vi "Log In.vi"(0 "SLSC Remote in":refnum<class "SLSC Remote.lvclass">, 1 "username":string, 2 "password":string, 5 "chassis":refnum<k21>, 11 "error in (no error)":errorcluster, 12 "connect timeout (60 sec)":dbl=60.0, 13 "save credentials to disk? (F)":bool) -> (4 "SLSC Remote out":refnum<class "SLSC Remote.lvclass">, 15 "error out":errorcluster)   [LabVIEW 2015, in "SLSC Interfaces.lvlib" / "SLSC Remote.lvclass"]
uses:
  SLSC Remote.lvclass
  <vilib>/NI/NI JSONRPC Server Framework/Classes/Server/JSONRPC Server.lvclass
  <vilib>/rajsite/i3-json/i3-json.lvlib
  <vilib>/rajsite/i3-json/JSON Generation/Create Value Files/Create Value - Object.vi
  <vilib>/rajsite/i3-json/JSON Generation/Add Object Parameter Files/Add Object Parameter - String.vi
  <vilib>/httpClient/LabVIEWHTTPClient.lvlib
  <vilib>/NI/NI JSONRPC Server Framework/Classes/Server/Format Client Request (Auto-Increment).vi
  <vilib>/httpClient/POSTBuffer.vi
  <vilib>/rajsite/i3-json/JSON Generation/Add Object Parameter Files/Add Object Parameter - Numeric.vi
  <vilib>/rajsite/i3-json/JSON Generation/Add Object Parameter Files/Add Object Parameter - Boolean.vi
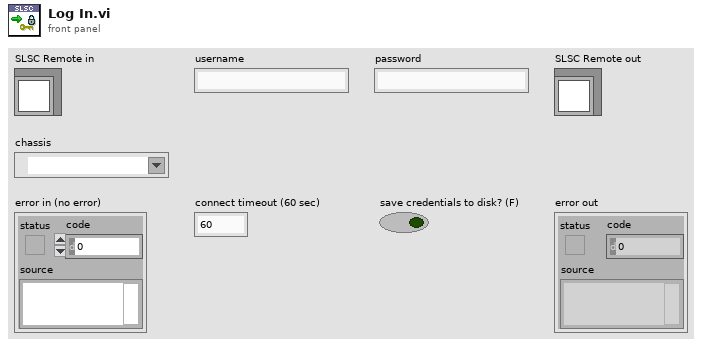
[diagram p1: front panel]
types:
  T1 = typedef "LabVIEWHTTPClient.lvlib/ClientHandle.ctl" = refnum<k1>
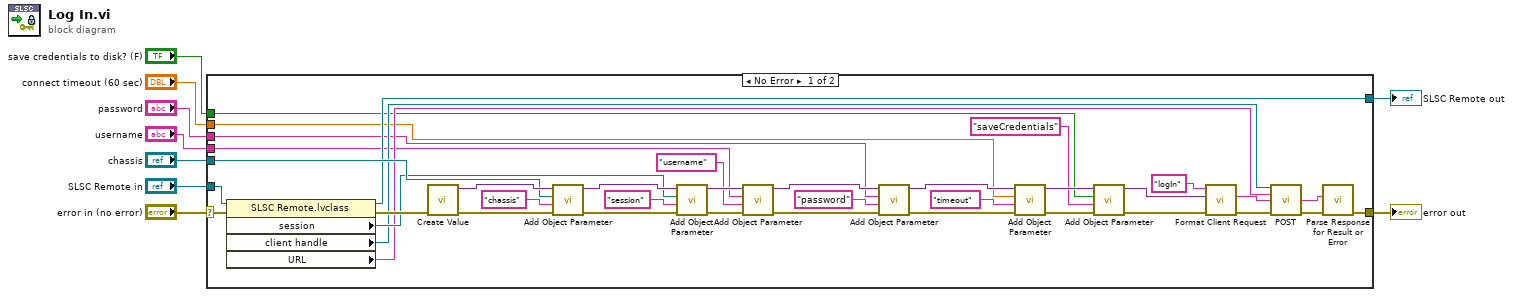
[diagram p0: block diagram]
diagram:
  n1 = case shown="No Error" "error in (no error)" {
    selector: "error in (no error)" -> [w42 w48]
    tunnel: "chassis" -> [w46 _]
    tunnel: "SLSC Remote in" -> [w44 w49]
    tunnel: [w43 w49] -> w5
    tunnel: [w28 w48] -> w6
    tunnel: "username" -> [w22 _]
    tunnel: "password" -> [w20 _]
    tunnel: "connect timeout (60 sec)" -> [w16 _]
    tunnel: "save credentials to disk? (F)" -> [w12 _]
    frame No Error {
      n2 = property class="SLSC Remote.lvclass"(reference=w44, error in=w42) -> (reference out=w43:refnum<class "SLSC Remote.lvclass">, error out=w41:errorcluster, "session"=w35:refnum<k21>, "client handle"=w33:T1, "URL"=w32:string)
      n3 = call-poly <vilib>:"Create Value.vi"("error in (no error)"=w41) -> ("error out"=w40:errorcluster, "JSON Tree"=w47:variant)  [unwired: 9 in]
      n4 = call-poly <vilib>:"Add Object Parameter.vi"("error in (no error)"=w40, "Name"="chassis", "String"=w46, "JSON Tree in (JSON Object)"=w47) -> ("error out"=w39:errorcluster, "JSON Tree out (JSON Object)"=w36:variant)  [unwired: 6 in]
      n5 = call-poly <vilib>:"Add Object Parameter.vi"("error in (no error)"=w39, "Name"="session", "String"=w35, "JSON Tree in (JSON Object)"=w36) -> ("error out"=w27:errorcluster, "JSON Tree out (JSON Object)"=w26:variant)  [unwired: 6 in]
      n6 = call-poly <vilib>:"Add Object Parameter.vi"("error in (no error)"=w27, "Name"="username" ("String"), "String"=w22, "JSON Tree in (JSON Object)"=w26) -> ("error out"=w25:errorcluster, "JSON Tree out (JSON Object)"=w24:variant)  [unwired: 6 in]
      n7 = call-poly <vilib>:"Add Object Parameter.vi"("error in (no error)"=w25, "Name"="password", "String"=w20, "JSON Tree in (JSON Object)"=w24) -> ("error out"=w19:errorcluster, "JSON Tree out (JSON Object)"=w18:variant)  [unwired: 6 in]
      n8 = call-poly <vilib>:"Add Object Parameter.vi"("error in (no error)"=w19, "Name"="timeout", "Numeric"=w16, "JSON Tree in (JSON Object)"=w18) -> ("error out"=w15:errorcluster, "JSON Tree out (JSON Object)"=w14:variant)  [unwired: 6 in]
      n9 = call-poly <vilib>:"Add Object Parameter.vi"("error in (no error)"=w15, "Name"="saveCredentials", "Boolean"=w12, "JSON Tree in (JSON Object)"=w14) -> ("error out"=w10:errorcluster, "JSON Tree out (JSON Object)"=w11:variant)  [unwired: 6 in]
      n10 = call-poly <vilib>:"Format Client Request.vi"("error in (no error)"=w10, "params"=w11, "method"="logIn") -> ("error out"=w31:errorcluster, "Request String"=w37:string)  [unwired: 7 in]
      n11 = call-poly <vilib>:"POST.vi"("client handle"=w33, "url"=w32, "buffer"=w37, "error in (no error)"=w31) -> ("body"=w30:string, "error out"=w29:errorcluster)  [unwired: 8 in, 2 out]
      n12 = call <vilib>:"Parse Response for Result or Error.vi"("error in"=w29, "Response String In"=w30) -> ("error out"=w28:errorcluster)  [unwired: 7 in, 2 out]
    }
    frame Error {
    }
  }
  "error out" <- w6
  "SLSC Remote out" <- w5
